vi "check_max_greater_or_equal_than_min.vi"(8 "max_len_in":u8, 11 "min_len_in":u8) -> (0 "max_len_out":i8, 3 "min_len_out":i8)   [LabVIEW 2024]
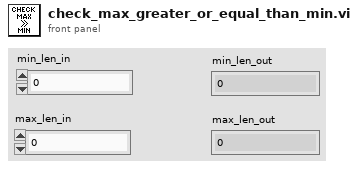
[diagram p1: front panel]
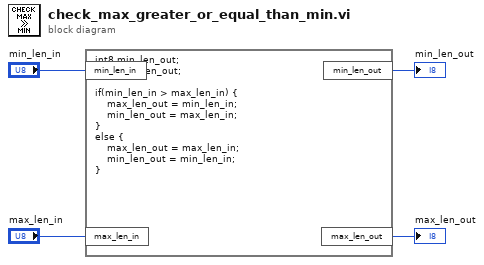
[diagram p0: block diagram]
diagram:
  n1 = formula code="int8 min_len_out;\nint8 max_len_out;\n\nif(min_len_in > max_len_in) {\n    max_len_out = min_len_in;\n    min_len_out = max_len_in;\n}\nelse {\n    max_len_out = max_len_in;\n    min_len_out = min_len_in;\n}"("max_len_in"="max_len_in", "min_len_in"="min_len_in") -> ("min_len_out"=→"min_len_out":i8, "max_len_out"=→"max_len_out":i8)
